vi "OW Read Bytes.vi"(7 "ReadDataLen":u32, 9 "pReadData":u8[](array[numeric])=array[4097 elements], 10 "ChannelMask":u32, 11 "DevHandle":i32) -> (1 "pReadData out":u8[](array[numeric]), 3 "function return":i32)   [LabVIEW 2010, in "usb2ow.lvlib"]
doc: "int WINAPI OW_ReadBytes(int DevHandle, unsigned int ChannelMask,unsigned char *pReadData,unsigned int ReadDataLen);"
uses:
  usb2ow.lvlib
  USB2XXX/trunk/USB2XXX/USB2XXX/vs2010/Release/USB2XXX.dll
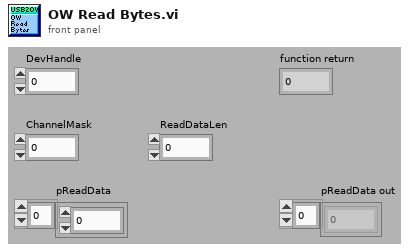
[diagram p1: front panel]
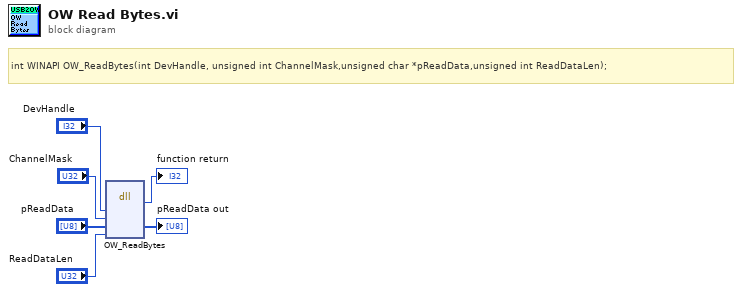
[diagram p0: block diagram]
diagram:
  # "int WINAPI OW_ReadBytes(int DevHandle, unsigned int ChannelMask,unsigned char *pReadData,unsigned int ReadDataLen);"
  n1 = dll-call lib="E:/OtherWork/STM32/USB2XXX/trunk/USB2XXX/USB2XXX/vs2010/Release/USB2XXX.*" fn="OW_ReadBytes"("DevHandle"="DevHandle", "ChannelMask"="ChannelMask", "pReadData"="pReadData", "ReadDataLen"="ReadDataLen") -> (→"function return":i32, "pReadData"=→"pReadData out":u8[])  [unwired: 6 in, 2 out]
